vi "StellarNet User Set Coefficients.vi"(10 "Channel":u8, 11 "Array":T1(array[cluster])=[{"Default Value"=0.718, "Description"="C1"}, {"Default Value"=0.00062, "Description"="C2"}, {"Default Value"=200.0, "Description"="C3"}, {"Default Value"=0.0, "Description"="C4"}]) -> (3 "Coeffs":dbl[](array[numeric]))   [LabVIEW 2023]
panel:
  in  "Continue":bool
  in  "Value":dbl
  out "Instruction":string
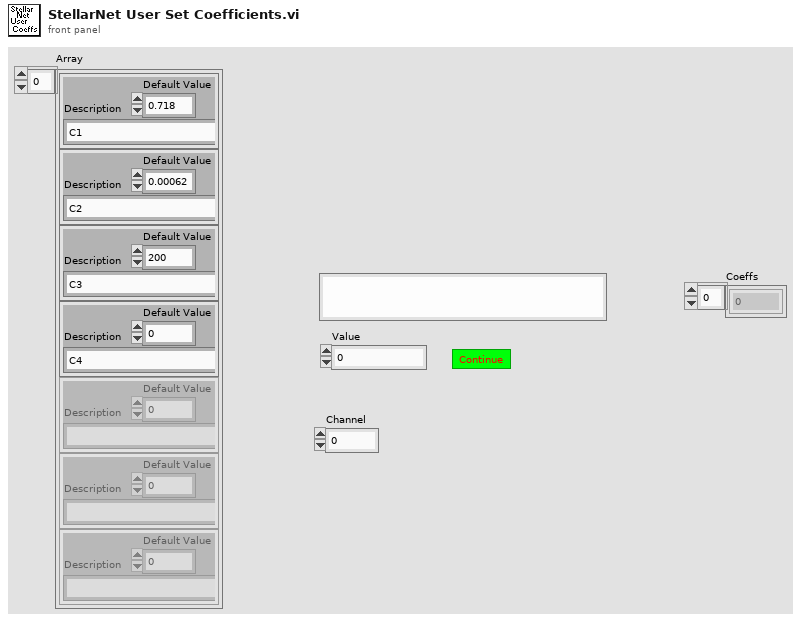
[diagram p1: front panel]
types:
  T1 = cluster{"Default Value":dbl, "Description":string}[]
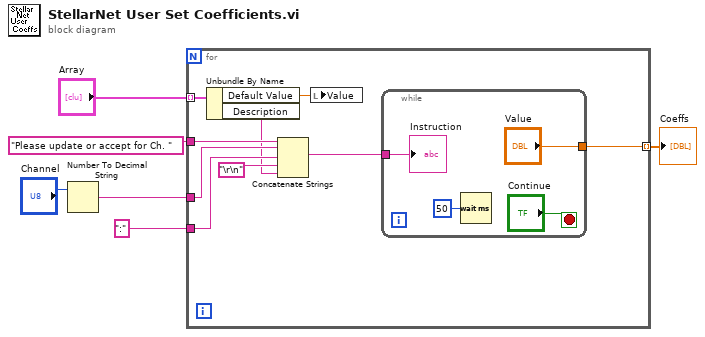
[diagram p0: block diagram]
diagram:
  n1 = Number To Decimal String(number="Channel") -> (decimal integer string=w2:string)  [unwired: 1 in]
  n2 = for {
    tunnel: "Array" -> [w15] mode=indexing
    tunnel: "Please update or accept for Ch. " -> [w13]
    tunnel: [w11] -> w4 mode=indexing
    tunnel: w2 -> [w10]
    tunnel: ":" -> [w9]
    n3 = Unbundle By Name(w15) -> ("Default Value"=w14:dbl, "Description"=w7:string)
    n4 = Concatenate Strings(w13, w10, w9, "\r\n", w7) -> (w12:string)
    n5 = local write "Value"(w14) -> ()
    n6 = while {
      tunnel: w12 -> [w18]
      tunnel: ["Value"] -> w11
      stop <- "Continue" stop-if-true
      n7 = Wait (ms)(milliseconds to wait=u32 50) -> ()  [unwired: 1 out]
      "Instruction" <- w18
    }
  }
  "Coeffs" <- w4
